vi "RightMotors.vi"   [LabVIEW 2020]
uses:
  <vilib>/Rock Robotics/WPI/Utilities/WPI_GetSetVariantRefNum.vi
  GlobalRight.vi
types:
  T1 = typedef "WPI_JoystickDevRef.ctl" = cluster{"Device":T2}
  T2 = typedef "WPI_JoystickDeviceEnum.ctl" = enum16{"USB 0", "USB 1", "USB 2", "USB 3", "USB 4", "USB 5"}
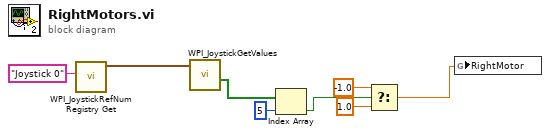
[diagram p0: block diagram]
diagram:
  n1 = call <vilib>:"WPI_JoystickRefNum Registry Get.vi"("refnum name"="Joystick 0") -> ("JoystickDevRef"=w8:T1)  [unwired: 9 in, 1 out]
  n2 = call <vilib>:"WPI_JoystickGetValues.vi"("JoystickDevRef"=w8) -> ("Buttons"=w6:bool[])  [unwired: 6 in, 4 out]
  n3 = Index Array(array=w6, index=5) -> (element=w4:bool)
  n4 = Select(t=-1.0, s=w4, f=1.0) -> (s? t:f=w1:dbl)
  n5 = global write "GlobalRight.vi" "RightMotor"(w1) -> ()
